vi "Slew Rate - Drive.vi"(4 "Slew Rate (Unit/Sec)":dbl, 6 "Disable Slew":bool, 9 "Right Motor Value":dbl, 10 "Left Motor Value":dbl) -> (1 "Right Motor Value":dbl, 2 "Left Motor Value":dbl)   [LabVIEW 2015]
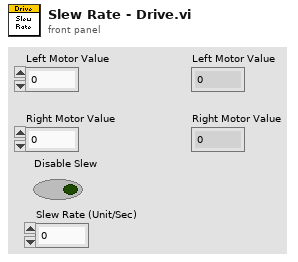
[diagram p1: front panel]
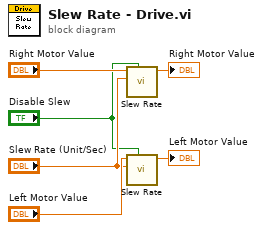
[diagram p0: block diagram]
diagram:
  n1 = call "Slew Rate.vi"("Disable"="Disable Slew", "Units / Second"="Slew Rate (Unit/Sec)", "Input"="Right Motor Value") -> ("Output"=→"Right Motor Value":dbl)  [unwired: 6 in, 2 out]
  n2 = call "Slew Rate.vi"("Disable"="Disable Slew", "Units / Second"="Slew Rate (Unit/Sec)", "Input"="Left Motor Value") -> ("Output"=→"Left Motor Value":dbl)  [unwired: 6 in, 2 out]
